vi "Init.vi"(8 "error in (no error)":errorcluster, 11 "Nestle Actor in":refnum<class "Nestle Actor.lvclass">) -> (0 "error out":errorcluster, 3 "Nestle Actor out":refnum<class "Nestle Actor.lvclass">)   [LabVIEW 2020, in "Nestle Actor.lvlib" / "Nestle Actor.lvclass"]
uses:
  Nestle Actor.lvclass
  Nestle Actor.lvclass/Nestle Actor.ctl
  <vilib>/Utility/config.llb/Read Key (Double).vi
  <vilib>/Utility/config.llb/Read Key (String).vi
  <vilib>/Utility/config.llb/NI_LVConfig.lvlib
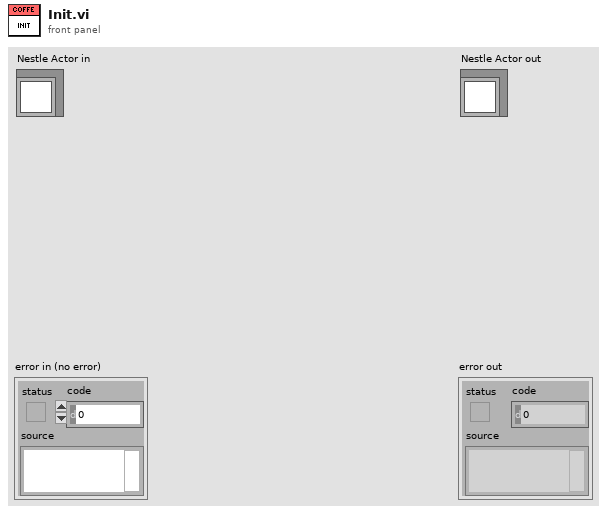
[diagram p1: front panel]
types:
  T1 = typedef "NI_LVConfig.lvlib/Config Data RefNum.ctl" = refnum<k1>
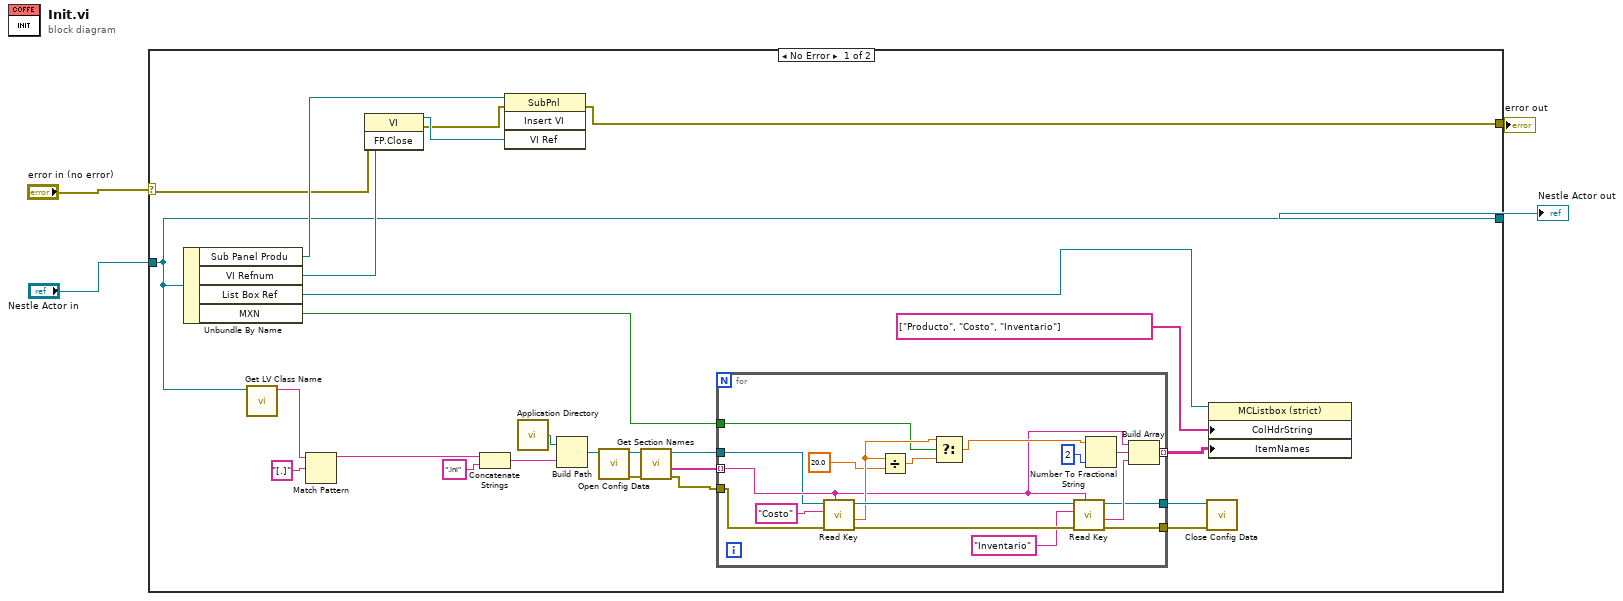
[diagram p0: block diagram]
diagram:
  n1 = case shown="No Error" "error in (no error)" {
    selector: "error in (no error)" -> [w25 w49]
    tunnel: [w24 w49] -> w3
    tunnel: [w23 w48] -> w1
    tunnel: "Nestle Actor in" -> [w23 w48]
    frame No Error {
      n2 = Unbundle By Name(w23) -> ("Sub Panel Produ"=w29:refnum<vi>, "VI Refnum"=w28:refnum<vi>, "List Box Ref"=w14:refnum<vi>, "MXN"=w6:bool)
      n3 = call <vilib>:"Get LV Class Name.vi"("object"=w23) -> ("class name"=w5:string)  [unwired: 9 in, 1 out]
      n4 = Match Pattern(string=w5, regular expression="[.]") -> (before substring=w17:string)  [unwired: 1 in, 3 out]
      n5 = invoke class="VI" method="FP.Close"(reference=w28, error in=w25) -> (reference out=w27:refnum<vi>, error out=w26:errorcluster)  [unwired: 1 in, 1 out]
      n6 = Concatenate Strings(w17, ".ini") -> (w21:string)
      n7 = invoke class="SubPnl" method="Insert VI"(reference=w29, error in=w26, "VI Ref"=w27) -> (error out=w24:errorcluster)  [unwired: 1 in, 3 out]
      n8 = call <vilib>:"Application Directory.vi"() -> ("Application Directory"=w22:path)
      n9 = Build Path(base path=w22, name or relative path=w21) -> (appended path=w19:path)
      n10 = call <vilib>:"Open Config Data.vi"("configuration file path"=w19) -> ("error out"=w15:errorcluster, "refnum"=w16:T1)  [unwired: 8 in, 1 out]
      n11 = call <vilib>:"Get Section Names.vi"("error in (no error)"=w15, "refnum"=w16) -> ("error out"=w9:errorcluster, "section names"=w11:string[], "refnum out"=w10:T1)  [unwired: 7 in]
      n12 = for {
        tunnel: [w36] -> w13 mode=indexing
        tunnel: w11 -> [w35] mode=indexing
        tunnel: w10 -> [w34]
        tunnel: w9 -> [w33]
        tunnel: [w32] -> w8
        tunnel: [w31] -> w7
        tunnel: w6 -> [w30]
        n13 = call-poly <vilib>:"Read Key.vi"("section"=w35, "error in (no error)"=w33, "key"="Costo", "refnum"=w34) -> ("error out"=w47:errorcluster, "value"=w38:dbl, "refnum out"=w46:T1)  [unwired: 4 in, 1 out]
        n14 = Divide(x=w38, y=20.0) -> (x/y=w39:dbl)
        n15 = Select(t=w38, s=w30, f=w39) -> (s? t:f=w40:dbl)
        n16 = call-poly <vilib>:"Read Key.vi"("section"=w35, "error in (no error)"=w47, "key"="Inventario", "refnum"=w46) -> ("error out"=w31:errorcluster, "value"=w43:string, "refnum out"=w32:T1)  [unwired: 4 in, 1 out]
        n17 = Number To Fractional String(number=w40, precision (6)=i16 2) -> (F-format string=w42:string)  [unwired: 2 in]
        n18 = Build Array(w35, w42, w43) -> (w36:string[])
      }
      n19 = call <vilib>:"Close Config Data.vi"("error in (no error)"=w7, "refnum"=w8) -> ()  [unwired: 8 in, 2 out]
      n20 = property class="MCListbox (strict)"(reference=w14, "ColHdrString"=string[] ["Producto", "Costo", "Inventario"] ("Column Header Strings[]"), "ItemNames"=w13) -> ()  [unwired: 1 in, 2 out]
    }
    frame Error {
    }
  }
  "error out" <- w3
  "Nestle Actor out" <- w1
